vi "GC_GaN.vi"() -> ()   [LabVIEW 2011]
uses:
  GlobalVariables.vi
panel:
  in  "stop":bool
  out "PP Rout":string="Pump Purge Rout"
  out "shutter_indicator":string
  in  "32":bool
  in  "91":bool
  in  "92":bool
  in  "97":bool
  in  "101":bool
  in  "108":bool
  in  "123":bool
  out "val102 2":bool
  in  "Fout25":dbl min=0.0 max=5000.0 format="%.1f"
  in  "Fout29":dbl min=0.0 max=5000.0 format="%.1f"
  in  "Fout30":dbl min=0.0 max=5000.0 format="%.1f"
  in  "Fout26":dbl min=0.0 max=5000.0 format="%.1f"
  in  "Fout52":dbl min=0.0 max=5000.0 format="%.1f"
  in  "Fout53":dbl min=0.0 max=5000.0 format="%.1f"
  in  "Fout54":dbl min=0.0 max=5000.0 format="%.1f"
  in  "Fout38":dbl min=0.0 max=5000.0 format="%.1f"
  in  "Fout41":dbl min=0.0 max=5000.0 format="%.1f"
  in  "Fout49":dbl min=0.0 max=5000.0 format="%.1f"
  in  "Fout50":dbl min=0.0 max=5000.0 format="%.1f"
  in  "Fout51":dbl min=0.0 max=5000.0 format="%.1f"
  in  "Fout73":dbl min=0.0 max=5000.0 format="%.1f"
  in  "Fout87":dbl min=0.0 max=5000.0 format="%.1f"
  in  "Fout84":dbl min=0.0 max=5000.0 format="%.1f"
  in  "Fout83":dbl min=0.0 max=5000.0 format="%.1f"
  in  "Fout88":dbl min=0.0 max=5000.0 format="%.1f"
  in  "Fout74":dbl min=0.0 max=5000.0 format="%.1f"
  in  "Fout75":dbl min=0.0 max=5000.0 format="%.1f"
  in  "Fout76":dbl min=0.0 max=5000.0 format="%.1f"
  in  "Fout85":dbl min=0.0 max=5000.0 format="%.1f"
  in  "Fout55":dbl min=0.0 max=5000.0 format="%.1f"
  out "Fin84":dbl format="%.1f"
  out "Fin88":dbl format="%.1f"
  out "Fin83":dbl format="%.1f"
  out "Fin87":dbl format="%.1f"
  out "Fin86":dbl format="%.1f"
  out "Fin85":dbl format="%.1f"
  out "Fin92":dbl format="%.1f"
  out "Fin93":dbl format="%.1f"
  out "Fin94":dbl format="%.1f"
  out "Fin60":dbl format="%.3e"
  out "Fin61":dbl format="%.3e"
  out "Fin65":dbl format="%.1f"
  out "Fin73":dbl format="%.1f"
  out "Fin66":dbl format="%.1f"
  out "Fin67":dbl format="%.1f"
  out "Fin68":dbl format="%.1f"
  out "Fin69":dbl format="%.1f"
  out "Fin70":dbl format="%.1f"
  out "Fin74":dbl format="%.1f"
  out "Fin75":dbl format="%.1f"
  out "Fin76":dbl format="%.1f"
  out "Fin27":dbl format="%.1f"
  out "Fin29 2":dbl format="%.1f"
  out "Fin30 2":dbl format="%.1f"
  out "Fin38 2":dbl format="%.1f"
  out "Fin42 2":dbl format="%.1f"
  out "Fin52":dbl format="%.1f"
  out "Fin53":dbl format="%.1f"
  out "Fin54":dbl format="%.1f"
  out "Fin43":dbl format="%.1f"
  out "Fin41 2":dbl format="%.1f"
  out "Fin25 2":dbl format="%.1f"
  out "Fin26 2":dbl format="%.1f"
  out "Fin40":dbl format="%.1f"
  out "Fin49":dbl format="%.1f"
  out "Fin50":dbl format="%.1f"
  out "Fin51":dbl format="%.1f"
  out "Fin28":dbl format="%.1f"
  out "Fin55":dbl format="%.1f"
  in  "110":bool caption="104"
  in  "111":bool
  in  "104":bool caption="110"
  in  "109":bool
  in  "112":bool
  in  "54":bool
  out "bub8":string="TMAl #2"
  out "bub7":string="TMGa"
  out "bub6":string="TEGa"
  out "bub5":string="TMIn #2"
  out "bub4":string="TMIn #1"
  out "bub3":string="TMAl #1"
  out "bub2":string="Cp2Mg"
  out "bub1":string="DEZn"
  out "gas2":string="SiH4"
  in  "37":bool
  in  "38":bool
  in  "34":bool
  in  "36":bool
  in  "33":bool
  in  "35":bool
  in  "43":bool
  out "Vac lock":string="locked"
  out "LL lock":string="locked"
  out "GV lock":string="locked"
  in  "50":bool
  in  "49":bool
  out "LL Door":bool
  in  "44":bool
  in  "46":bool
  in  "40":bool
  in  "56":bool
  in  "42":bool
  in  "93":bool
  in  "39":bool
  in  "41":bool
  in  "47":bool
  in  "26":bool
  in  "53":bool
  in  "45":bool
  in  "55":bool
  in  "GV Down":bool=TRUE
  in  "GV Up":bool
  in  "30":bool
  in  "31":bool
  in  "94":bool
  in  "51":bool
  in  "103":bool
  in  "48":bool
  in  "28":bool
  in  "val102":bool
  in  "52":bool
  # "102"
  # "102"
  # "INNER"
  # "INNER"
  # "MIDDLE"
  # "MIDDLE"
  # "OUTER"
  # "OUTER"
  # "VOLTAGE"
  # "VOLTAGE"
  # "CURRENT"
  # "CURRENT"
  # "POWER"
  # "POWER"
  # "VIEW PORT\n   SHIELD"
  # "VIEW PORT\n   SHIELD"
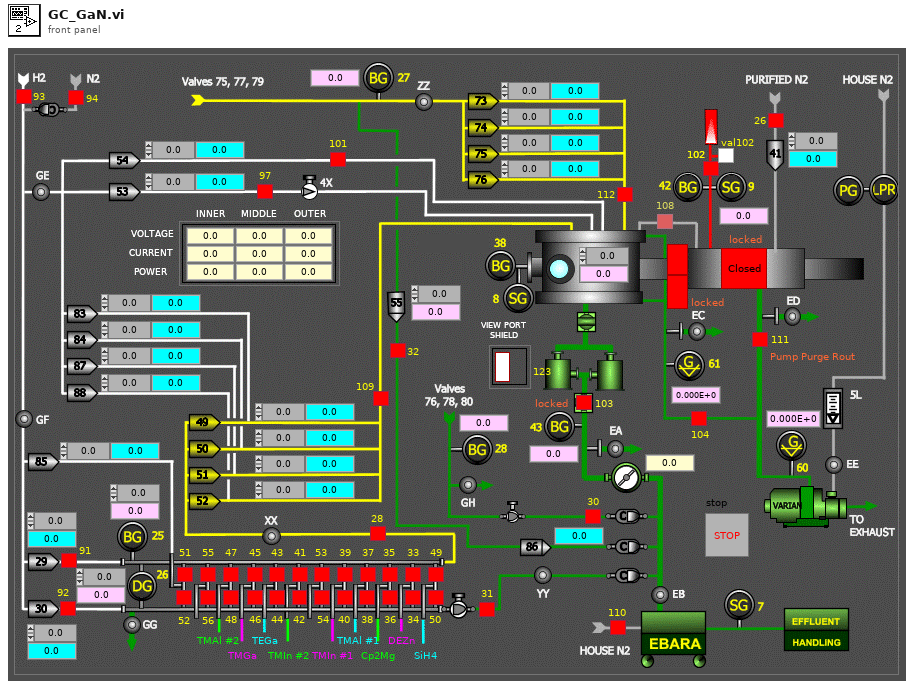
[diagram p1: front panel]
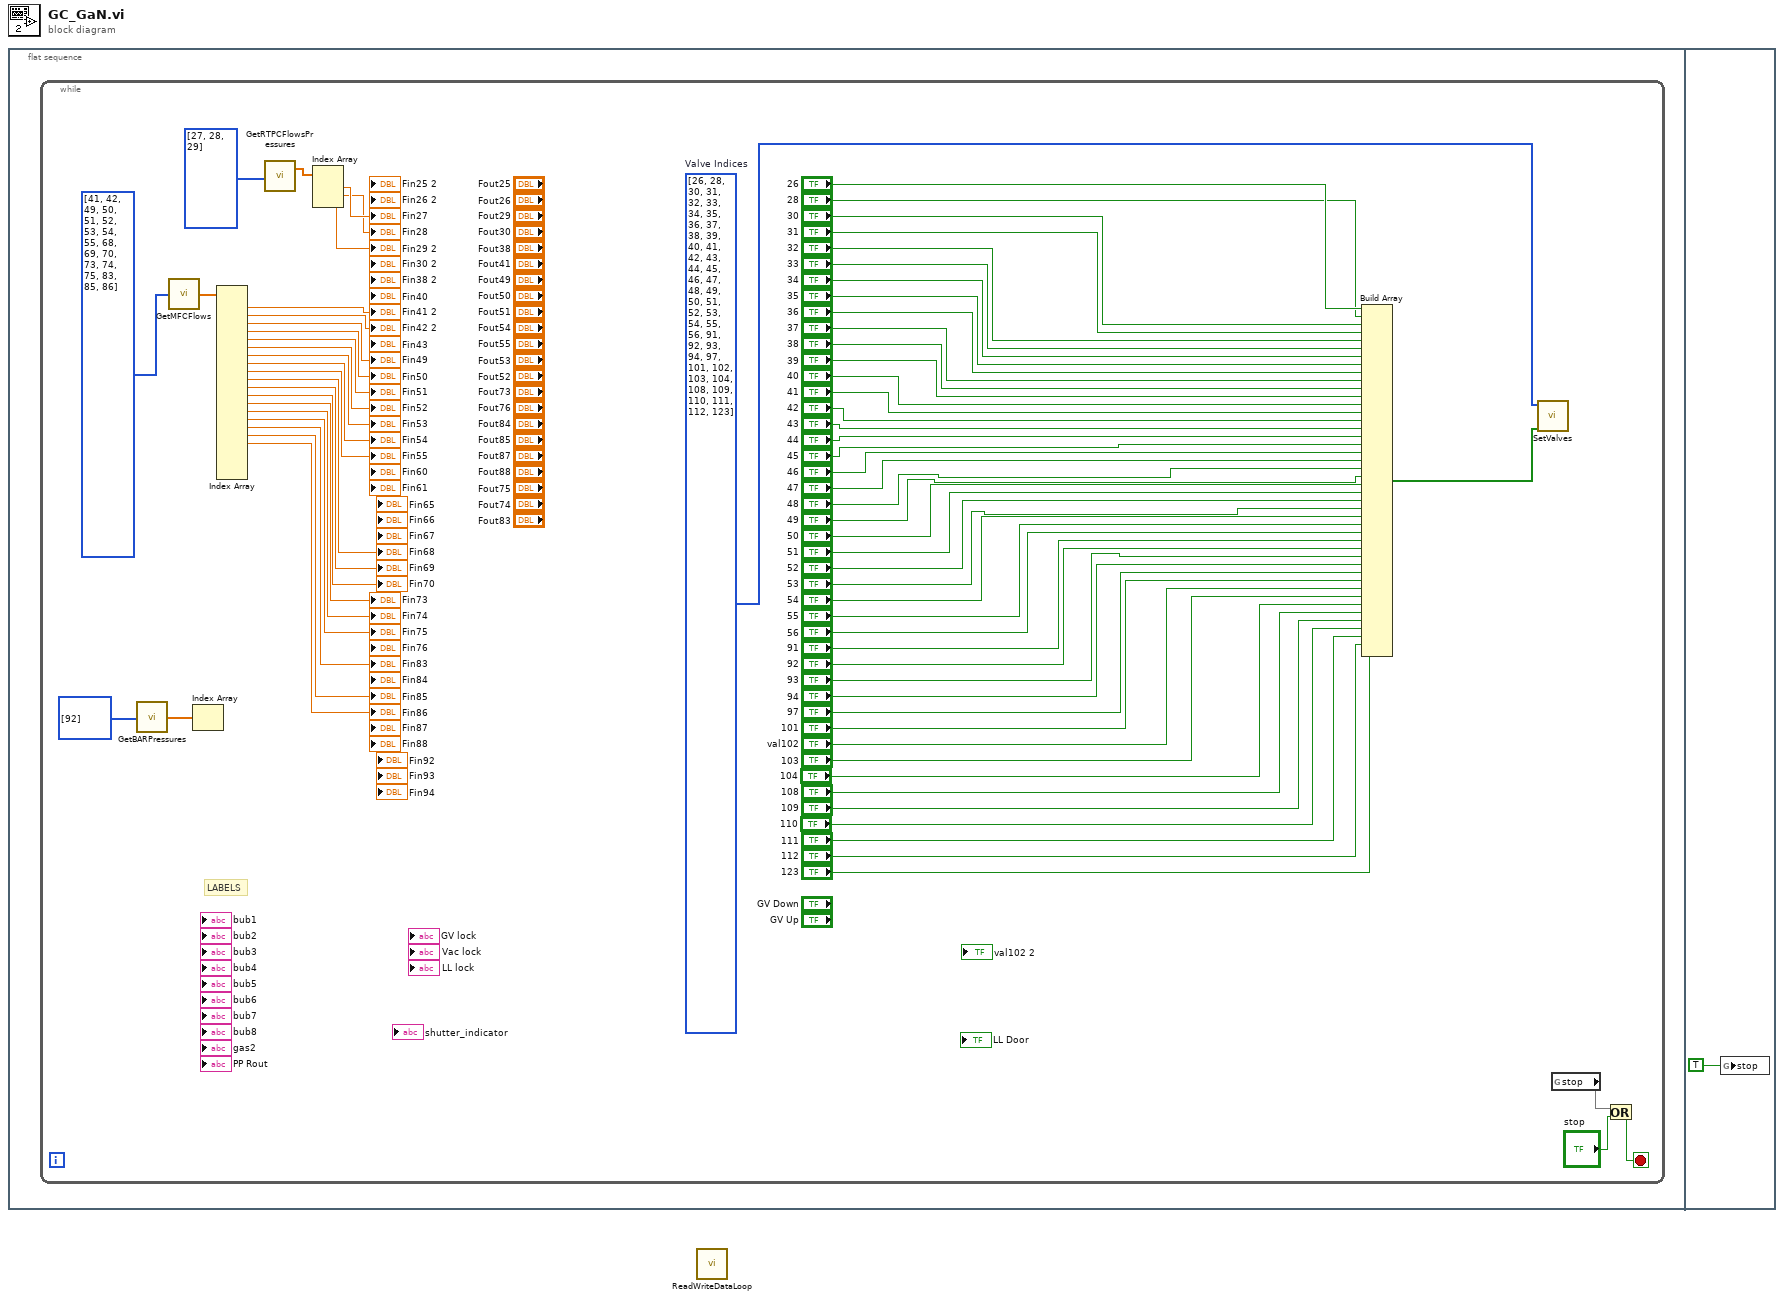
[diagram p0: block diagram]
diagram:
  n1 = flat-sequence {
    frame #0 {
      n2 = while {
        stop <- w30 stop-if-true
        w34 = i32[] [26, 28, 30, 31, 32, 33, 34, 35, 36, 37, 38, 39, 40, 41, 42, 43, 44, 45, 46, 47, 48, 49, 50, 51, 52, 53, 54, 55, 56, 91, 92, 93, 94, 97, 101, 102, 103, 104, 108, 109, 110, 111, 112, 123]  # Valve Indices
        # "LABELS"
        n3 = call "GetBARPressures.vi"("BAR Indices"=i32[] [92]) -> ("Pressures"=w3:dbl[])
        n4 = call "GetMFCFlows.vi"("Indices"=i32[] [41, 42, 49, 50, 51, 52, 53, 54, 55, 68, 69, 70, 73, 74, 75, 83, 85, 86]) -> ("Flows"=w28:dbl[])
        n5 = Index Array(array=w3) -> ()  [unwired: 1 in, 1 out]
        n6 = Index Array(array=w28) -> (element #1=→"Fin41 2":dbl, element #2=→"Fin42 2":dbl, element #3=→"Fin49":dbl, element #4=→"Fin50":dbl, element #5=→"Fin51":dbl, element #6=→"Fin52":dbl, element #7=→"Fin53":dbl, element #8=→"Fin54":dbl, element #9=→"Fin55":dbl, element #10=→"Fin68":dbl, element #11=→"Fin69":dbl, element #12=→"Fin70":dbl, element #13=→"Fin73":dbl, element #14=→"Fin74":dbl, element #15=→"Fin75":dbl, element #16=→"Fin83":dbl, element #17=→"Fin85":dbl, element #18=→"Fin86":dbl)  [unwired: 22 in, 4 out]
        n7 = call "GetRTPCFlowsPressures.vi"("Indices"=i32[] [27, 28, 29]) -> ("Flows"=w8:dbl[])  [unwired: 1 out]
        n8 = Index Array(array=w8) -> (element #1=→"Fin27":dbl, element #2=→"Fin28":dbl, element #3=→"Fin29 2":dbl)  [unwired: 3 in]
        n9 = Build Array("26", "28", "30", "31", "32", "33", "34", "35", "36", "37", "38", "39", "40", "41", "42", "43", "44", "45", "46", "47", "48", "49", "50", "51", "52", "53", "54", "55", "56", "91", "92", "93", "94", "97", "101", "val102", "103", "104", "108", "109", "110", "111", "112", "123") -> (w33:bool[])
        n10 = call "SetValves.vi"("Boolean Array"=w33, "Indices"=w34) -> ()  [unwired: 10 in]
        n11 = global read "GlobalVariables.vi" "stop"() -> (w31)
        n12 = Or(x=w31, y="stop") -> (x .or. y?=w30:bool)
      }
    }
    frame #1 {
      n13 = global write "GlobalVariables.vi" "stop"(TRUE ("stop")) -> ()
    }
  }
  n14 = call "ReadWriteDataLoop.vi"() -> ()  [unwired: 11 in, 1 out]
